vi "Control Descriptions Updater.vi"() -> ()   [LabVIEW 2017]
panel:
  out "Rest of Input String":string
  in  "JSON Items":string[](array[string])
  in  "Item Names":string[](array[string])
  out "Offset past":i32 caption="Offset past Value"
  in  "Section Name (Cluster Name)":string
  in  "JSON Sections":string="{}"
  in  "enable LabVIEW extensions? (T)":bool=TRUE
  in  "Data Type and Default Value":variant
  in  "Anything":variant
  out "Item Names":string[](array[string])
  out "Item offset":i32
  out "Item Offsets":i32[](array[numeric])
  in  "Pretty Print?":bool
  out "<JSON>":string
  in  "$Path":string
  in  "$Path or Item Name":string
  in  "JSON":string
  in  "Offset":i32
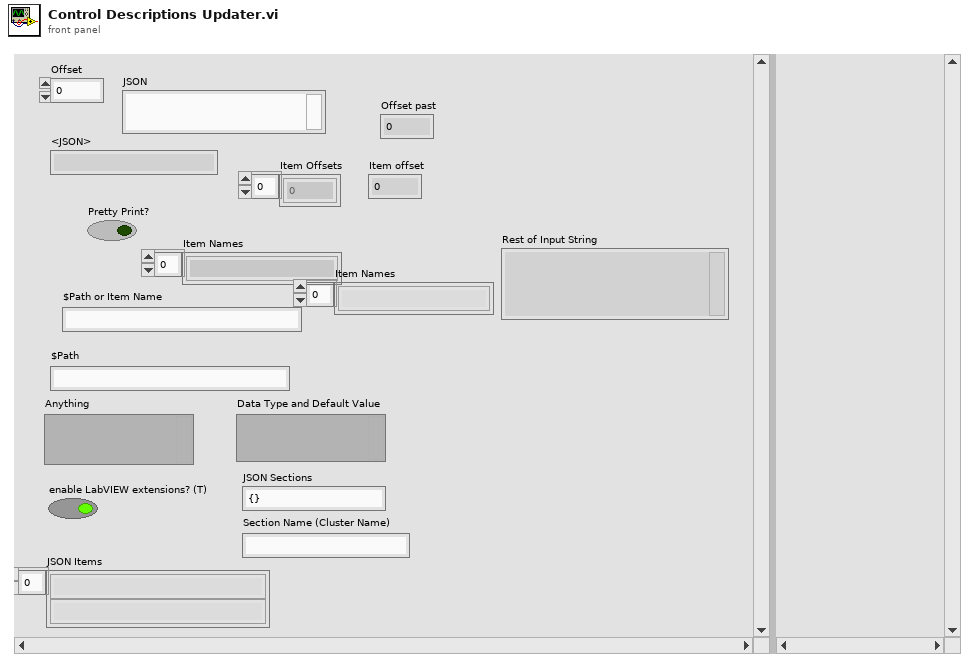
[diagram p1: front panel]
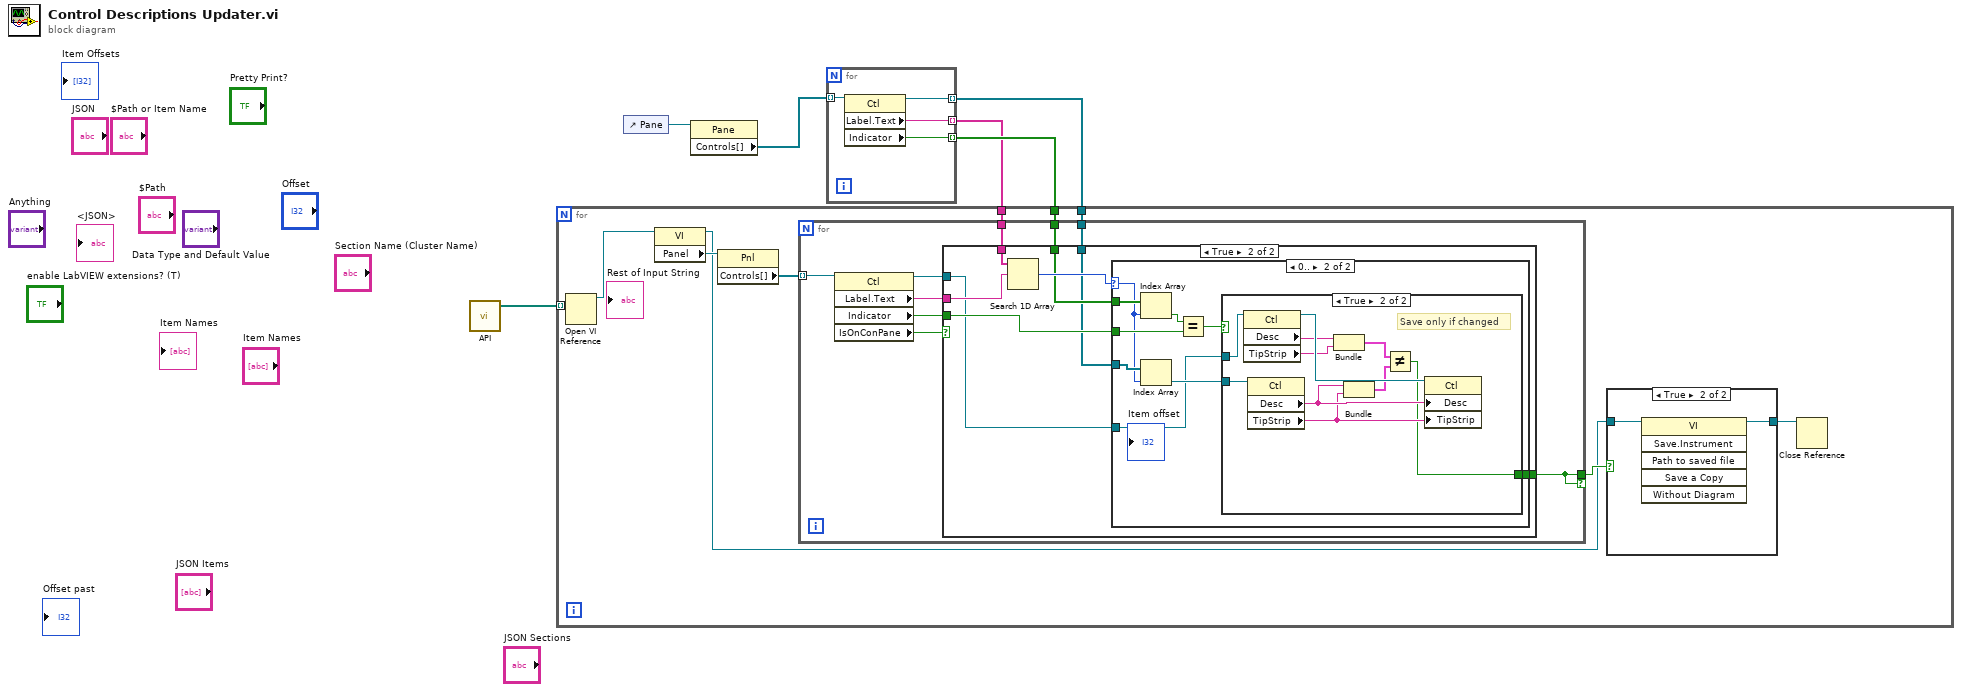
[diagram p0: block diagram]
diagram:
  n1 = call "API.vi"() -> ("API"=w6:path[])  [unwired: 9 in, 2 out]
  n2 = control-ref of="Pane"() -> (w5:refnum<vi>)
  n3 = property class="Pane"(reference=w5) -> ("Controls[]"=w4:refnum<vi>[])  [unwired: 1 in, 2 out]
  n4 = for {
    tunnel: w4 -> [w10] mode=indexing
    tunnel: [w9] -> w2 mode=indexing
    tunnel: [w8] -> w3 mode=indexing
    tunnel: [w7] -> w1 mode=indexing
    n5 = property class="Ctl"(reference=w10) -> (reference out=w7:refnum<vi>, "Label.Text"=w9:string, "Indicator"=w8:bool)  [unwired: 1 in, 1 out]
  }
  n6 = for {
    tunnel: w6 -> [w18] mode=indexing
    tunnel: w3 -> [w16]
    tunnel: w2 -> [w15]
    tunnel: w1 -> [w14]
    n7 = Open VI Reference(vi path=w18) -> (vi reference=w17:refnum<vi>)  [unwired: 5 in, 1 out]
    n8 = property class="VI"(reference=w17) -> (reference out=w12:refnum<vi>, "Panel"=w20:refnum<vi>)  [unwired: 1 in, 1 out]
    n9 = property class="Pnl"(reference=w20) -> ("Controls[]"=w19:refnum<vi>[])  [unwired: 1 in, 2 out]
    n10 = for {
      tunnel: w19 -> [w32] mode=indexing
      tunnel: w15 -> [w31]
      tunnel: w16 -> [w29]
      tunnel: w14 -> [w26]
      tunnel: [w24] -> w13 if=w24
      n11 = property class="Ctl"(reference=w32) -> (reference out=w25:refnum<vi>, "Label.Text"=w30:string, "Indicator"=w28:bool, "IsOnConPane"=w27:bool)  [unwired: 1 in, 1 out]
      n12 = case shown="True" w27 {
        tunnel: w31 -> [_ w40]
        tunnel: w30 -> [_ w39]
        tunnel: w29 -> [_ w37]
        tunnel: w28 -> [_ w36]
        tunnel: w26 -> [_ w35]
        tunnel: w25 -> [_ w34]
        tunnel: [_ w33] -> w24
        frame False {
        }
        frame True {
          n13 = Search 1D Array(1D array=w40, element=w39) -> (index of element=w38:i32)  [unwired: 1 in]
          n14 = case shown="0.." w38 {
            selector: w38 -> [_ w44]
            tunnel: w37 -> [_ w49]
            tunnel: w36 -> [_ w47]
            tunnel: w35 -> [_ w45]
            tunnel: w34 -> [_ w42]
            tunnel: [_ w41] -> w33
            frame ..-1 {
            }
            frame 0.. {
              n15 = Index Array(array=w49, index=w44) -> (element=w48:bool)
              n16 = Index Array(array=w45, index=w44) -> (element=w43:refnum<vi>)
              n17 = Equal?(x=w48, y=w47) -> (x = y?=w46:bool)
              n18 = case shown="True" w46 {
                tunnel: w43 -> [_ w59]
                tunnel: w42 -> [_ w58]
                tunnel: [_ w50] -> w41
                frame False {
                }
                frame True {
                  # "Save only if changed"
                  n19 = property class="Ctl"(reference=w58) -> (reference out=w57:refnum<vi>, "Desc"=w56:string, "TipStrip"=w55:string)  [unwired: 1 in, 1 out]
                  n20 = property class="Ctl"(reference=w59) -> ("Desc"=w54:string, "TipStrip"=w53:string)  [unwired: 1 in, 2 out]
                  n21 = Bundle("Desc"=w56, "TipStrip"=w55) -> (w52:cluster{"Desc":string, "TipStrip":string})  [unwired: 1 in]
                  n22 = Bundle("Desc"=w54, "TipStrip"=w53) -> (w51:cluster{"Desc":string, "TipStrip":string})  [unwired: 1 in]
                  n23 = Not Equal?(x=w52, y=w51) -> (x != y?=w50:bool)
                  n24 = property class="Ctl"(reference=w57, "Desc"=w54, "TipStrip"=w53) -> ()  [unwired: 1 in, 2 out]
                }
              }
            }
          }
        }
      }
    }
    n25 = case shown="True" w13 {
      tunnel: w12 -> [w21 w23]
      tunnel: [w21 w22] -> w11
      frame False {
      }
      frame True {
        n26 = invoke class="VI" method="Save.Instrument"(reference=w23) -> (reference out=w22:refnum<vi>)  [unwired: 5 in, 5 out]
      }
    }
    n27 = Close Reference(reference=w11) -> ()  [unwired: 1 in, 1 out]
  }
